vi "Read Ref.vi"(8 "error in (no error)":errorcluster, 11 "VISA in":refnum<class "VISA.lvclass">) -> (0 "error out":errorcluster, 2 "Ref":refnum<visa-resource-name>, 3 "VISA out":refnum<class "VISA.lvclass">)   [LabVIEW 2018, in "Protocols.lvlib" / "VISA.lvclass"]
uses:
  VISA.lvclass
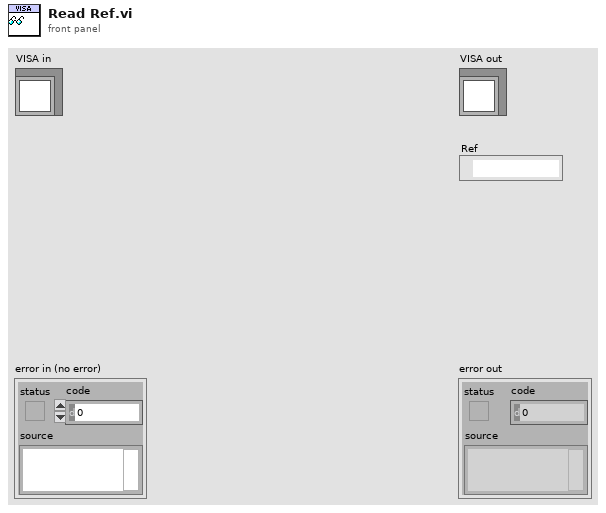
[diagram p1: front panel]
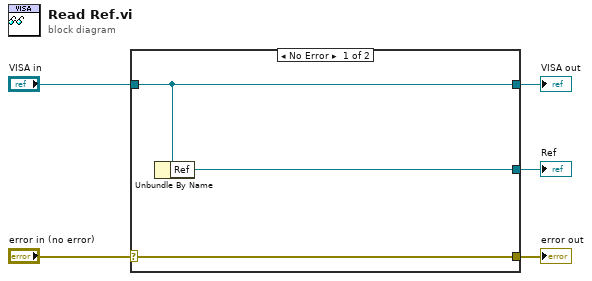
[diagram p0: block diagram]
diagram:
  n1 = case shown="No Error" "error in (no error)" {
    selector: "error in (no error)" -> [w8 w9]
    tunnel: [w8 w9] -> w4
    tunnel: [w7 w10] -> w2
    tunnel: "VISA in" -> [w7 w10]
    tunnel: [w6 _] -> w1
    frame No Error {
      n2 = Unbundle By Name(w7) -> ("Ref"=w6:refnum<visa-resource-name>)
    }
    frame Error {
    }
  }
  "error out" <- w4
  "VISA out" <- w2
  "Ref" <- w1
